vi "test Send Terminate.vi"(8 "error in":errorcluster) -> (0 "error out":errorcluster)   [LabVIEW 2020, in "serenial.io-ase.test.lvlib"]
uses:
  serenial.io-ase.test.lvlib
  serenial.io-ase/ase/Call State.ctl
  serenial.io-ase/ase/ase.lvclass/ase.ctl
  serenial.io-ase/ase/Start Call (Exe Path).vi
  serenial.io-ase/ase/Start Call (Exe Name).vi
  serenial.io-ase/ase/Merge Call Library Errors.vi
  serenial.io-ase/ase/Error Invalid ASE Handle.vi
  serenial.io-ase/ase/Error Empty Executable Name.vi
  serenial.io-ase/ase/Check Shared Library Version.vi
  <vilib>/dlg_ctls.llb/Space Constant.vi
  serenial.io-ase/ase/Error Internal Library Implementation Error.vi
  <vilib>/Utility/file.llb/Application Directory.vi
  <vilib>/Utility/error.llb/Error Cluster From Error Code.vi
  <vilib>/addons/_JKI Toolkits/Caraya/classes/Assert/Assert Not Error.vi
  <vilib>/addons/_JKI Toolkits/Caraya/classes/Assert/Assert Not Equal Value and Type_Variant.vi
  <vilib>/addons/_JKI Toolkits/Caraya/classes/Assert/Assert Equal Value and Type_Variant.vi
  serenial.io-ase/configuration/configuration.lvclass
  serenial.io-ase/ase/ase.lvclass
  <vilib>/addons/_JKI Toolkits/Caraya/classes/Assert/Assert.lvclass
  <vilib>/addons/_JKI Toolkits/Caraya/classes/Test/Test.lvclass
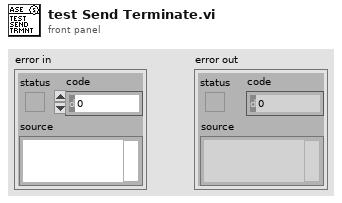
[diagram p1: front panel]
types:
  T1 = typedef "serenial.io-ase.lvlib/ase.lvclass/Call State.ctl" = enum16{"Running/Terminating", "Already Exited"}
  T2 = typedef "serenial.io-ase.lvlib/ase.lvclass/Event References.ctl" = cluster{"Standard Output":refnum<user-event>, "Standard Error":refnum<user-event>, "Did Exit":refnum<user-event>}
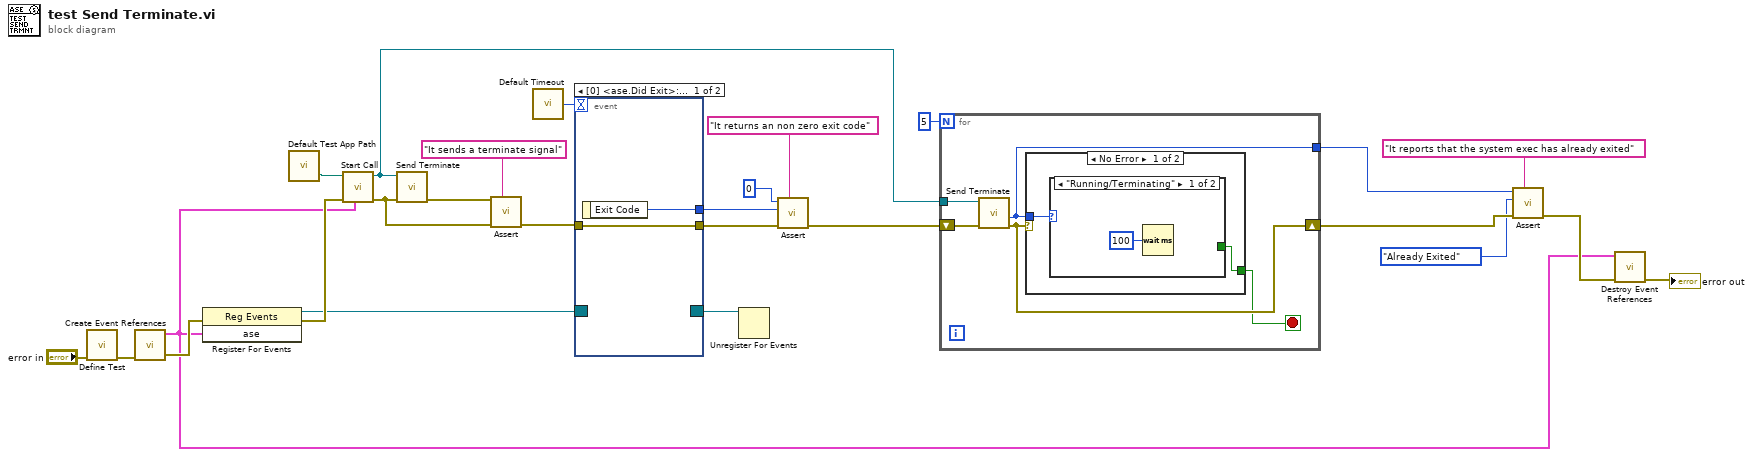
[diagram p0: block diagram]
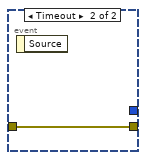
[diagram p2: hidden frame]
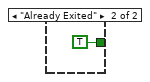
[diagram p3: hidden frame]
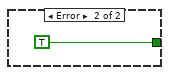
[diagram p4: hidden frame]
diagram:
  n1 = call <vilib>:"Define Test.vi"("error in (no error)"="error in") -> ("error out"=w25:errorcluster)  [unwired: 10 in]
  n2 = call "Create Event References.vi"("error in"=w25) -> ("error out"=w26:errorcluster, "ase"=w6:T2)  [unwired: 9 in]
  n3 = register-events(error in=w26, w6) -> (reference out=w20:refnum<event-registration>, error out=w21:errorcluster)  [unwired: 1 in]
  n4 = call "Default Test App Path.vi"() -> ("Exe Path"=w1:path)  [unwired: 2 in, 1 out]
  n5 = call-poly "Start Call.vi"("Event References"=w6, "error in"=w21, "Executable Path"=w1) -> ("error out"=w3:errorcluster, "New ASE Handle"=w7:refnum<class "ase.lvclass">)  [unwired: 7 in]
  n6 = call "Send Terminate.vi"("error in"=w3, "ASE Handle"=w7) -> ("error out"=w4:errorcluster)  [unwired: 7 in, 2 out]
  n7 = call-poly <vilib>:"Assert.vi"("Label"="It sends a terminate signal", "error in (no error)"=w3, "Not Error?"=w4) -> ("error out"=w14:errorcluster)  [unwired: 8 in]
  n8 = call "Default Timeout.vi"() -> ("Default Timeout"=w9:i32)
  n9 = event shown="[0] <ase.Did Exit>: User Event" {
    selector: w20 -> [_ _]
    dyn-events: [_ _] -> w23
    timeout: w9 -> [_ _]
    tunnel: w14 -> [w27 w29]
    tunnel: [w27 w29] -> w19
    tunnel: [w28 _] -> w18
    event User Event {
      n10 = event-data() -> ("Exit Code"=w28:i32)  [unwired: 1 in]
    }
    event Timeout {
      n11 = event-data() -> ()  [unwired: 1 in, 1 out]
    }
  }
  n12 = Unregister For Events(event registration refnum=w23) -> ()  [unwired: 1 in, 1 out]
  n13 = call-poly <vilib>:"Assert.vi"("Label"="It returns an non zero exit code", "error in (no error)"=w19, "Y"=w18, "X"=i64 0 ("Exit Code")) -> ("error out"=w8:errorcluster)  [unwired: 7 in]
  n14 = for {
    N: 5 -> [_]
    tunnel: [w31] -> w13
    tunnel: w7 -> [w33]
    shift-right: [w32] -> w12
    shift-left: w8 -> [w34]
    stop <- w30 stop-if-true
    n15 = call "Send Terminate.vi"("error in"=w34, "ASE Handle"=w33) -> ("error out"=w32:errorcluster, "State"=w31:T1)  [unwired: 7 in, 1 out]
    n16 = case shown="No Error" w32 {
      tunnel: w31 -> [w36 _]
      tunnel: [w35 TRUE] -> w30
      frame No Error {
        n17 = case shown="\"Running/Terminating\"" w36 {
          tunnel: [_ TRUE] -> w35
          frame "Running/Terminating" {
            n18 = Wait (ms)(milliseconds to wait=u32 100) -> ()  [unwired: 1 out]
          }
          frame "Already Exited" {
          }
        }
      }
      frame Error {
      }
    }
  }
  n19 = call-poly <vilib>:"Assert.vi"("Label"="It reports that the system exec has already exited", "error in (no error)"=w12, "Y"=Call_State."Already Exited" ("State"), "X"=w13) -> ("error out"=w11:errorcluster)  [unwired: 7 in]
  n20 = call "Destroy Event References.vi"("error in"=w11, "Event References"=w6) -> ("error out"=→"error out":errorcluster)  [unwired: 9 in]
